vi "PPG_ABC.calc channel times.vi"(0 "i ref in":refnum<vi>, 1 "channelTable":string[](array[string]), 2 "timeTable":dbl[](array[numeric]), 5 "error in (no error)":errorcluster) -> (14 "i ref out":refnum<vi>, 15 "channelTimes":dbl[][](array[numeric]), 19 "error out":errorcluster)   [LabVIEW 2014, in "PPG_ABC.lvlib"]
doc: "Calculates the output times of all channels of a configuration. At this point, the channels are not yet synchronized to each other. Please note, that the times given are absolute times and indicate when (!) and channel should switch (and not after which time it should switch)."
uses:
  PPG_ABC.lvlib
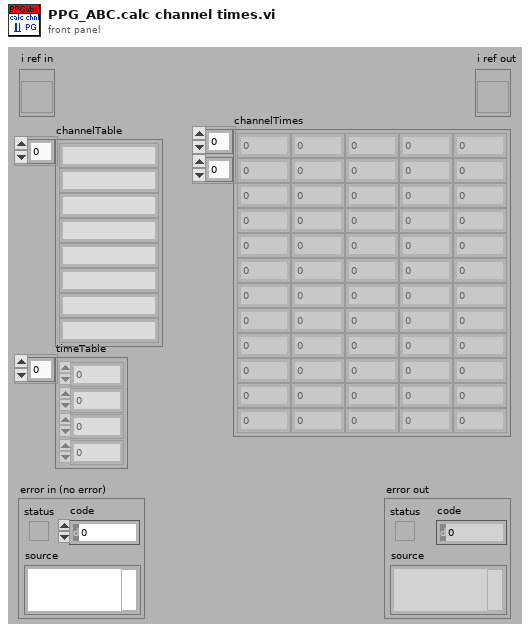
[diagram p1: front panel]
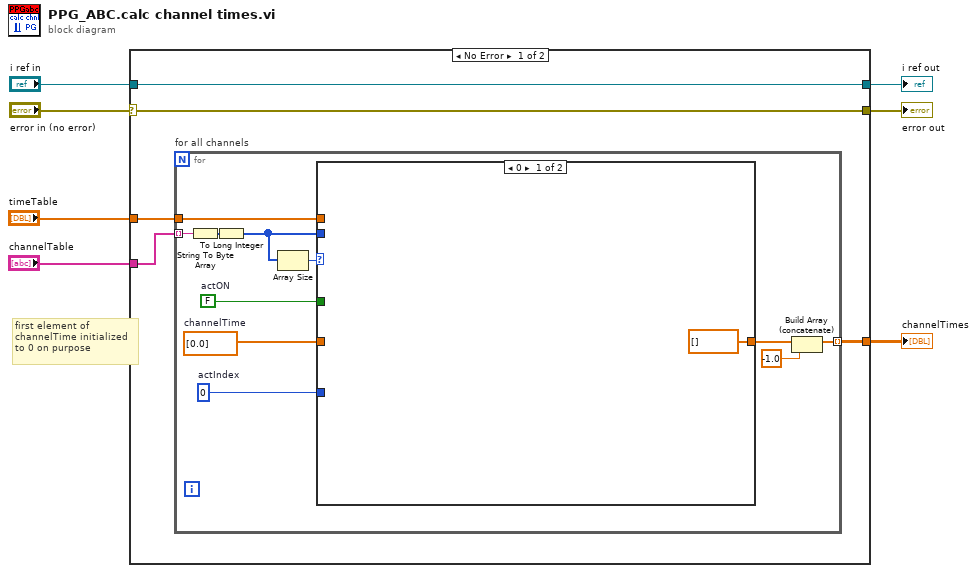
[diagram p0: block diagram]
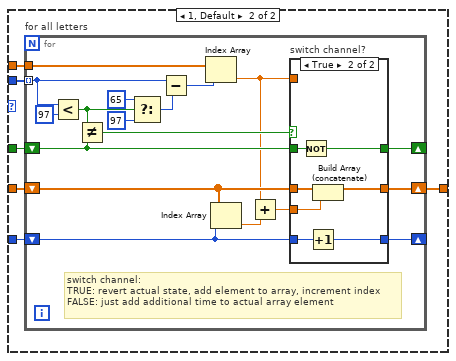
[diagram p2: hidden frame]
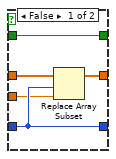
[diagram p3: hidden frame]
diagram:
  # "first element of \nchannelTime initialized\nto 0 on purpose"
  n1 = case shown="No Error" "error in (no error)" {
    selector: "error in (no error)" -> [w11 w61]
    tunnel: "i ref in" -> [w12 w62]
    tunnel: [w12 w62] -> w6
    tunnel: [w11 w61] -> w5
    tunnel: [w10 _] -> w1
    tunnel: "timeTable" -> [w9 _]
    tunnel: "channelTable" -> [w8 _]
    frame No Error {
      n2 = for "for all channels" {
        tunnel: w8 -> [w23] mode=indexing
        tunnel: w9 -> [w18]
        tunnel: [w15] -> w10 mode=indexing
        w19 = 0  # actIndex
        w20 = FALSE  # actON
        w21 = dbl[] [0.0]  # channelTime
        n3 = String To Byte Array(string=w23) -> (unsigned byte array=w22:u8[])
        n4 = To Long Integer(number=w22) -> (32bit integer=w14:i32[])
        n5 = Array Size(array=w14) -> (size(s)=w13:i32)
        n6 = case shown="0" w13 {
          tunnel: w21 -> [_ w30]
          tunnel: w20 -> [_ w29]
          tunnel: w19 -> [_ w28]
          tunnel: w18 -> [_ w27]
          tunnel: [dbl[] [] ("channelTime") w26] -> w17
          tunnel: w14 -> [_ w25]
          frame 0 {
          }
          frame 1, Default {
            n7 = for "for all letters" {
              tunnel: w25 -> [w43] mode=indexing
              shift-right: [w39] -> w26
              shift-left: w30 -> [w34]
              shift-right: [w36] -> _
              shift-left: w29 -> [w37]
              shift-right: [w38] -> _
              shift-left: w28 -> [w35]
              tunnel: w27 -> [w41]
              # "switch channel:\nTRUE: revert actual state, add element to array, increment index\nFALSE: just add additional time to actual array element"
              n8 = Less?(x=w43, y=97) -> (x < y?=w46:bool)
              n9 = Not Equal?(x=w46, y=w37) -> (x != y?=w47:bool)
              n10 = Select(t=65, s=w46, f=97) -> (s? t:f=w42:i32)
              n11 = Subtract(x=w43, y=w42) -> (x-y=w40:i32)
              n12 = Index Array(array=w41, index=w40) -> (element=w32:dbl)
              n13 = Index Array(array=w34, index=w35) -> (element=w33:dbl)
              n14 = Add(x=w32, y=w33) -> (x+y=w31:dbl)
              n15 = case "switch channel?" shown="True" w47 {
                tunnel: w34 -> [w53 w58]
                tunnel: w35 -> [w51 w60]
                tunnel: w32 -> [_ _]
                tunnel: [w52 w57] -> w39
                tunnel: [w51 w59] -> w38
                tunnel: w37 -> [w50 w56]
                tunnel: [w50 w55] -> w36
                tunnel: w31 -> [w49 w54]
                frame False {
                  n16 = Replace Array Subset(array=w53, new element=w49, index=w51) -> (w52:dbl[])
                }
                frame True {
                  n17 = Not(x=w56) -> (.not. x?=w55:bool)
                  n18 = Increment(x=w60) -> (x+1=w59:i32)
                  n19 = Build Array (concatenate)(w58, w54) -> (w57:dbl[])
                }
              }
            }
          }
        }
        n20 = Build Array (concatenate)(w17, -1.0) -> (w15:dbl[])
      }
    }
    frame Error {
    }
  }
  "error out" <- w5
  "i ref out" <- w6
  "channelTimes" <- w1
